vi "Files already exsist.vi"(8 "error in (no error)":errorcluster, 11 "Metadata in":string[][](array[string])) -> (0 "error out":errorcluster, 2 "Files already exsist":bool, 3 "Metadata out":string[][](array[string]))   [LabVIEW 2013]
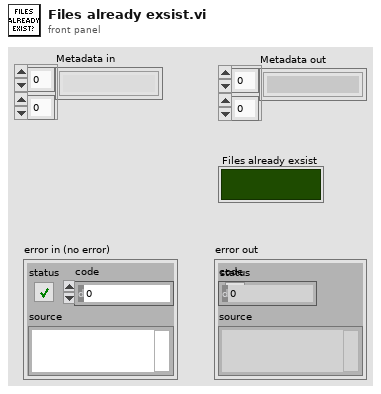
[diagram p1: front panel]
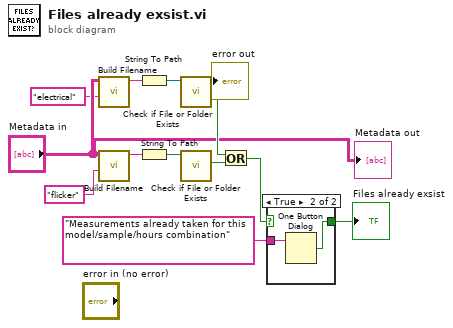
[diagram p0: block diagram]
diagram:
  n1 = call "Build Filename.vi"("Measurment Type"="electrical", "Metadata In"="Metadata in") -> ("String"=w4:string)  [unwired: 9 in]
  n2 = call "Build Filename.vi"("Measurment Type"="flicker", "Metadata In"="Metadata in") -> ("String"=w7:string)  [unwired: 9 in]
  n3 = String To Path(string=w4) -> (path=w5:path)
  n4 = String To Path(string=w7) -> (path=w6:path)
  n5 = call <vilib>:"Check if File or Folder Exists.vi"("path"=w5) -> ("file or folder exists?"=w8:bool)  [unwired: 8 in, 2 out]
  n6 = call <vilib>:"Check if File or Folder Exists.vi"("path"=w6) -> ("file or folder exists?"=w9:bool)  [unwired: 8 in, 2 out]
  n7 = Or(x=w8, y=w9) -> (x .or. y?=w10:bool)
  n8 = case shown="True" w10 {
    selector: w10 -> [w13 _]
    tunnel: [w13 w15] -> w11
    tunnel: "Measurements already taken for this model/sample/hours combination" -> [_ w14]
    frame False {
    }
    frame True {
      n9 = One Button Dialog(message=w14) -> (true=w15:bool)  [unwired: 1 in]
    }
  }
  "Files already exsist" <- w11
  "Metadata out" <- "Metadata in"
